vi "MostRecentHit.vi"(10 "Secondary hits":T2(array[cluster]), 11 "Primary hits":T1) -> (2 "NumofHits primaries":i32, 3 "Most recent hit":u64)   [LabVIEW 2016]
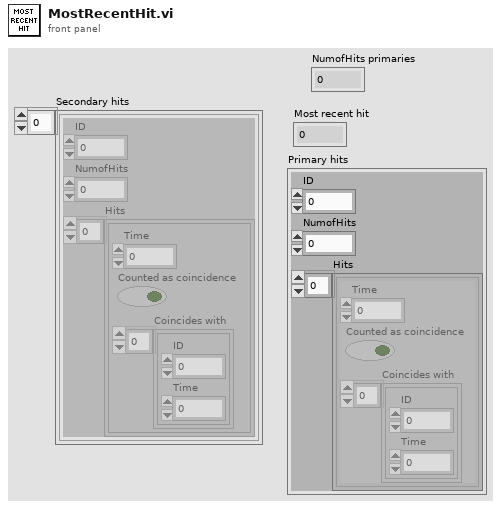
[diagram p1: front panel]
types:
  T1 = cluster{"ID":i8, "NumofHits":i32, "Hits":cluster{"Time":u64, "Counted as coincidence":bool, "Coincides with":cluster{"ID":i8, "Time":u64}[]}[]}
  T2 = cluster{"ID":i8, "NumofHits":i32, "Hits":cluster{"Time":u64, "Counted as coincidence":bool, "Coincides with":cluster{"ID":i8, "Time":u64}[]}[]}[]
  T3 = cluster{"Time":u64, "Counted as coincidence":bool, "Coincides with":cluster{"ID":i8, "Time":u64}[]}[]
  T4 = cluster{"Time":u64, "Counted as coincidence":bool, "Coincides with":cluster{"ID":i8, "Time":u64}[]}
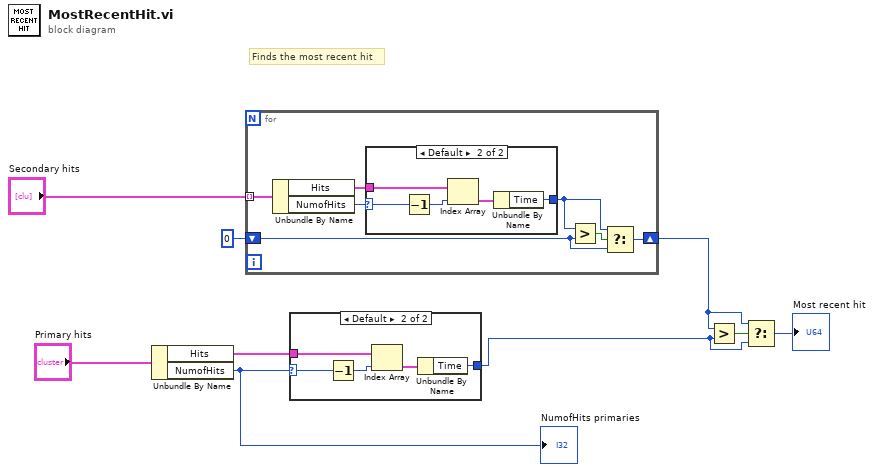
[diagram p0: block diagram]
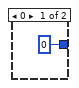
[diagram p2: hidden frame]
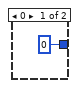
[diagram p3: hidden frame]
diagram:
  # "Finds the most recent hit"
  n1 = Unbundle By Name("Primary hits") -> ("Hits"=w7:T3, "NumofHits"=w6:i32)
  "NumofHits primaries" <- w6
  n2 = for {
    tunnel: "Secondary hits" -> [w16] mode=indexing
    shift-right: [w12] -> w3
    shift-left: u64 0 -> [w11]
    n3 = Unbundle By Name(w16) -> ("Hits"=w15:T3, "NumofHits"=w14:i32)
    n4 = case shown="Default" w14 {
      selector: w14 -> [_ w21]
      tunnel: w15 -> [_ w22]
      tunnel: [u64 0 ("Time") w18] -> w10
      frame 0 {
      }
      frame Default {
        n5 = Decrement(x=w21) -> (x-1=w20:i32)
        n6 = Index Array(array=w22, index=w20) -> (element=w19:T4)
        n7 = Unbundle By Name(w19) -> ("Time"=w18:u64)
      }
    }
    n8 = Greater?(x=w10, y=w11) -> (0:w13:bool)
    n9 = Select(t=w10, s=w13, f=w11) -> (s? t:f=w12:u64)
  }
  n10 = case shown="Default" w6 {
    selector: w6 -> [_ w27]
    tunnel: w7 -> [_ w28]
    tunnel: [u64 0 ("Time") w24] -> w2
    frame 0 {
    }
    frame Default {
      n11 = Decrement(x=w27) -> (x-1=w26:i32)
      n12 = Index Array(array=w28, index=w26) -> (element=w25:T4)
      n13 = Unbundle By Name(w25) -> ("Time"=w24:u64)
    }
  }
  n14 = Greater?(x=w3, y=w2) -> (0:w4:bool)
  n15 = Select(t=w3, s=w4, f=w2) -> (s? t:f=→"Most recent hit":u64)
